vi "Estimate_Across_Bivariate.vi"(8 "Estimation Ranges":T1={"Range mean X"={"Size"=8.0, "Min"=3.0, "Max/Step"=1.0, "Max (T) / Step (F)"=FALSE}, "Range mean Y"={"Size"=20.0, "Min"=1.0, "Max/Step"=0.5, "Max (T) / Step (F)"=FALSE}, "Range SD X"={"Size"=6.0, "Min"=0.5, "Max/Step"=0.5, "Max (T) / Step (F)"=FALSE}, "Range SD Y"={"Size"=6.0, "Min"=0.5, "Max/Step"=0.5, "Max (T) / Step (F)"=FALSE}}, 11 "Data":cluster{"X Sides":dbl, "Y Spacing":dbl}) -> (0 "A likelihoods, p(n,d|A)":dbl[][](graph)=[[0.06686866999999999, 0.08124426000000001, 0.06493801, 0.03670863, 0.011140430000000002], [0.08111895, 0.09855810000000001, 0.07877685000000001, 0.044531549999999996, 0.01351455], [0.06205023, 0.07538994, 0.060258690000000004, 0.03406347, 0.01033767], [0.03403664, 0.04135392, 0.03305392, 0.01868496, 0.005670560000000001], [0.012225509999999998, 0.01485378, 0.011872530000000001, 0.006711389999999999, 0.00203679]], 2 "4D Likelihoods":dbl[][][][](array[numeric]), 3 "Marginalize Across SD's":dbl[][](array[numeric]), 4 "output cluster":T2)   [LabVIEW 2017]
panel:
  out "N Calculations":i32
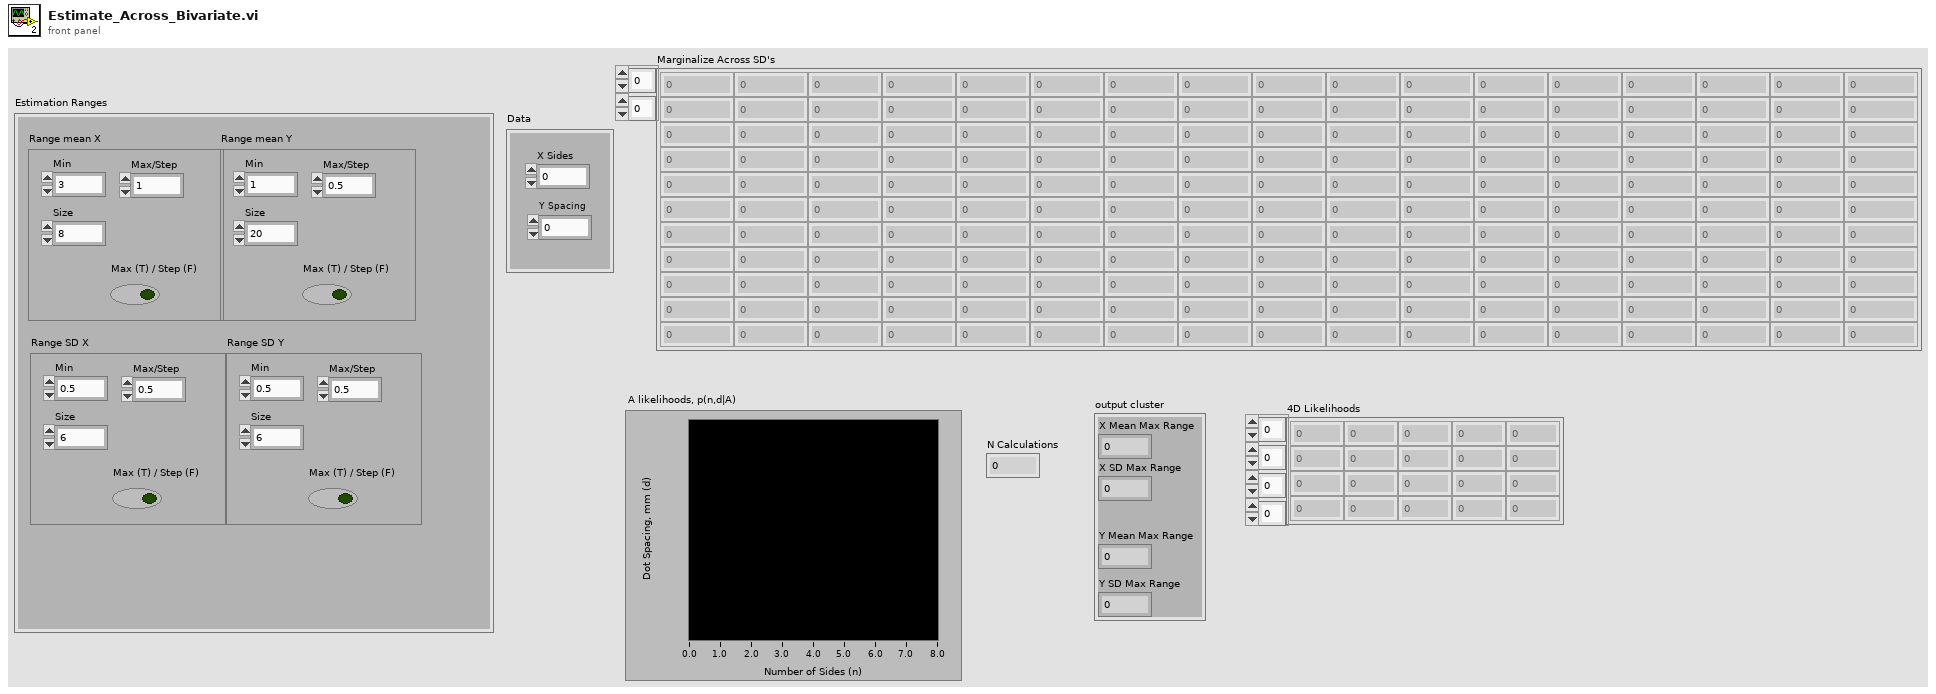
[diagram p1: front panel]
types:
  T1 = cluster{"Range mean X":cluster{"Size":dbl, "Min":dbl, "Max/Step":dbl, "Max (T) / Step (F)":bool}, "Range mean Y":cluster{"Size":dbl, "Min":dbl, "Max/Step":dbl, "Max (T) / Step (F)":bool}, "Range SD X":cluster{"Size":dbl, "Min":dbl, "Max/Step":dbl, "Max (T) / Step (F)":bool}, "Range SD Y":cluster{"Size":dbl, "Min":dbl, "Max/Step":dbl, "Max (T) / Step (F)":bool}}
  T2 = cluster{"X Mean Max Range":dbl, "X SD Max Range":dbl, "Y Mean Max Range":dbl, "Y SD Max Range":dbl}
  T3 = cluster{"Size":dbl, "Min":dbl, "Max/Step":dbl, "Max (T) / Step (F)":bool}
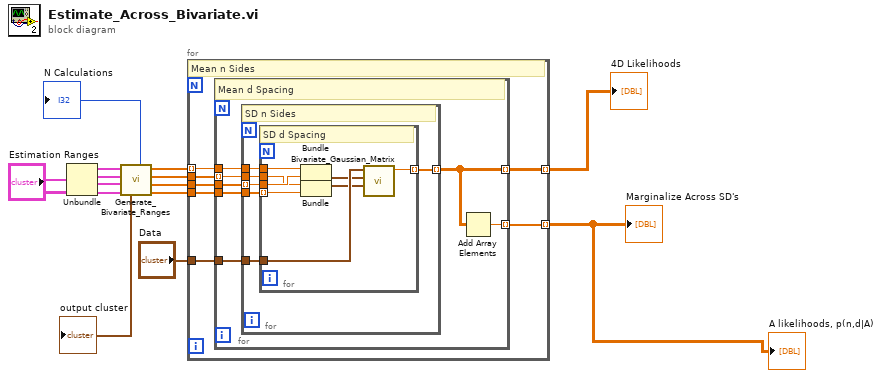
[diagram p0: block diagram]
diagram:
  n1 = Unbundle("Estimation Ranges") -> ("Range mean X"=w4:T3, "Range mean Y"=w3:T3, "Range SD X"=w2:T3, "Range SD Y"=w1:T3)
  n2 = call "Generate_Bivariate_Ranges.vi"("Range mean SD Y"=w1, "Range mean SD X"=w2, "Range mean Y"=w3, "Range mean X"=w4) -> ("Range SD B"=w14:dbl[], "Range SD A"=w9:dbl[], "Range Mean B"=w11:dbl[], "Range Mean A"=w10:dbl[], "N Calculations"=→"N Calculations":i32, "output cluster"=→"output cluster":T2)  [unwired: 2 in]
  n3 = for {
    tunnel: w10 -> [w21] mode=indexing
    tunnel: w9 -> [w20]
    tunnel: w11 -> [w19]
    tunnel: w14 -> [w18]
    tunnel: "Data" -> [w17]
    tunnel: [w16] -> w8 mode=indexing
    tunnel: [w15] -> w6 mode=indexing
    # "Mean n Sides"
    n4 = for {
      tunnel: w21 -> [w28]
      tunnel: w20 -> [w27]
      tunnel: w19 -> [w26] mode=indexing
      tunnel: w18 -> [w25]
      tunnel: w17 -> [w24]
      tunnel: [w23] -> w16 mode=indexing
      tunnel: [w22] -> w15 mode=indexing
      # "Mean d Spacing"
      n5 = for {
        tunnel: w28 -> [w34]
        tunnel: w27 -> [w33] mode=indexing
        tunnel: w26 -> [w32]
        tunnel: w25 -> [w31]
        tunnel: w24 -> [w30]
        tunnel: [w29] -> w23 mode=indexing
        # "SD n Sides"
        n6 = for {
          tunnel: w34 -> [w39]
          tunnel: w33 -> [w38]
          tunnel: w32 -> [w37]
          tunnel: w31 -> [w36] mode=indexing
          tunnel: w30 -> [w42]
          tunnel: [w35] -> w29 mode=indexing
          # "SD d Spacing"
          n7 = Bundle(w39, w38) -> (w41:cluster{dbl, dbl})  [unwired: 1 in]
          n8 = Bundle(w37, w36) -> (w40:cluster{dbl, dbl})  [unwired: 1 in]
          n9 = call "Bivariate_Gaussian_Matrix.vi"("B"=w40, "A"=w41, "Data"=w42) -> ("P"=w35:dbl)  [unwired: 5 in, 3 out]
        }
      }
      n10 = Add Array Elements(numeric array=w23) -> (sum=w22:dbl)
    }
  }
  "4D Likelihoods" <- w8
  "Marginalize Across SD's" <- w6
  "A likelihoods, p(n,d|A)" <- w6
